vi "init_waypoint.vi"(9 "No Sail Circles":T2[](array[typedef]), 10 "Coords":T1, 11 "Tolerance (meters?)":dbl) -> (3 "Waypoint out":refnum<class "Waypoint.lvclass">)   [LabVIEW 2011, in "Waypoint.lvclass"]
uses:
  Waypoint.lvclass
  2 Typedefs/UTM Circle.ctl
  2 Typedefs/UTM Location.ctl
panel:
  in  "Waypoint in":refnum<class "Waypoint.lvclass">
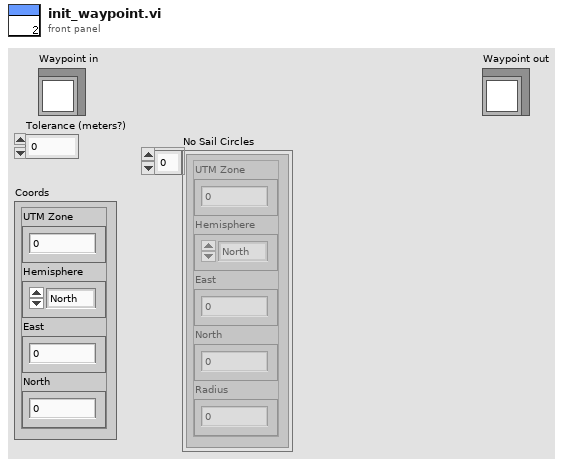
[diagram p1: front panel]
types:
  T1 = typedef "UTM Location.ctl" = cluster{"UTM Zone":dbl, "Hemisphere":enum16{"North", "South"}, "East":dbl, "North":dbl}
  T2 = typedef "UTM Circle.ctl" = cluster{"UTM Zone":dbl, "Hemisphere":enum16{"North", "South"}, "East":dbl, "North":dbl, "Radius":dbl}
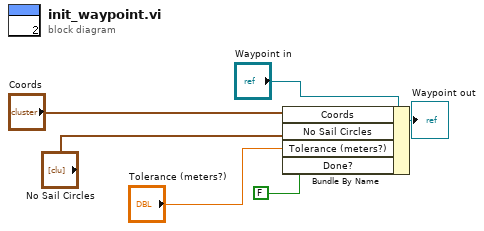
[diagram p0: block diagram]
diagram:
  n1 = Bundle By Name(cluster="Waypoint in", "Coords"="Coords", "No Sail Circles"="No Sail Circles", "Tolerance (meters?)"="Tolerance (meters?)", "Done?"=FALSE) -> (→"Waypoint out":refnum<class "Waypoint.lvclass">)
